vi "shutdownHW.vi"(8 "error in (no error)":errorcluster, 11 "Model in":refnum<class "Model.lvclass">) -> (0 "error out":errorcluster, 3 "Model out":refnum<class "Model.lvclass">)   [LabVIEW 2016, in "Model.lvclass"]
doc: "Shuts down the hardware."
uses:
  Model.lvclass
  Model.lvclass/Model.ctl
  Target/Target/Target.lvclass
  ss_sedspectrometer/SEDSpectrometer/SEDSpectrometer.lvclass
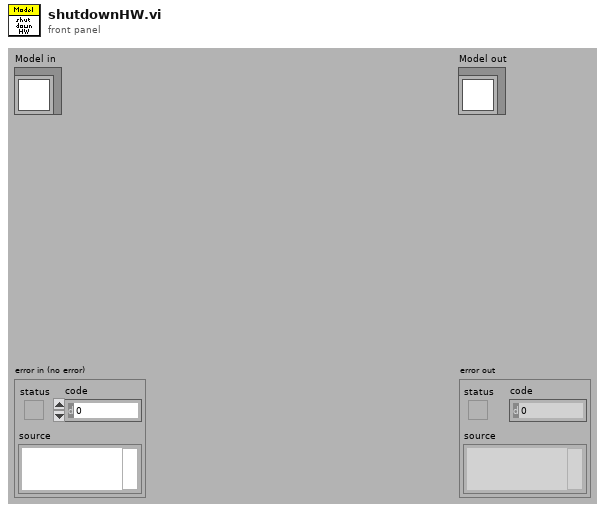
[diagram p1: front panel]
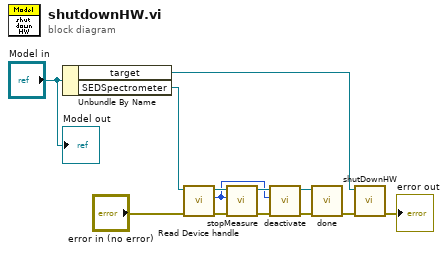
[diagram p0: block diagram]
diagram:
  n1 = Unbundle By Name("Model in") -> ("target"=w12:refnum<class "Target.lvclass">, "SEDSpectrometer"=w10:refnum<class "SEDSpectrometer.lvclass">)
  n2 = call-dynamic "Read Device handle.vi"("error in (no error)"="error in (no error)", "SEDSpectrometer in"=w10) -> ("error out"=w4:errorcluster, "Device handle"=w1:i32, "SEDSpectrometer out"=w3:refnum<class "SEDSpectrometer.lvclass">)  [unwired: 7 in]
  n3 = call "stopMeasure.vi"("error in (no error)"=w4, "Device"=w1, "SEDSpectrometer in"=w3) -> ("error out"=w5:errorcluster, "SEDSpectrometer out"=w2:refnum<class "SEDSpectrometer.lvclass">)  [unwired: 6 in, 1 out]
  n4 = call "deactivate.vi"("error in (no error)"=w5, "Handle"=w1, "SEDSpectrometer in"=w2) -> ("error out"=w6:errorcluster, "SEDSpectrometer out"=w7:refnum<class "SEDSpectrometer.lvclass">)  [unwired: 6 in, 1 out]
  n5 = call "done.vi"("error in (no error)"=w6, "SEDSpectrometer in"=w7) -> ("error out"=w8:errorcluster)  [unwired: 7 in, 2 out]
  n6 = call-dynamic "shutDownHW.vi"("error in (no error)"=w8, "Target in"=w12) -> ("error out"=→"error out":errorcluster)  [unwired: 8 in, 1 out]
  "Model out" <- "Model in"
